vi "InitSubChannel.vi"(9 "GUID":string, 10 "subchannel":i32, 11 "MessengerMCPU in":refnum<class "MessengerMCPU.lvclass">) -> (1 "GUIDsubchannel":i32, 3 "MessengerMCPU out":refnum<class "MessengerMCPU.lvclass">)   [LabVIEW 2019, in "MessengerM.lvlib" / "MessengerMCPU.lvclass"]
uses:
  MessengerMCPU.lvclass
  SubChannelCPU/SubChannelCPU.lvclass
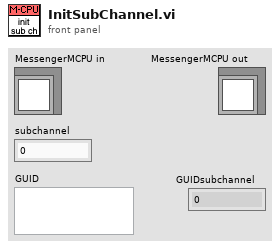
[diagram p1: front panel]
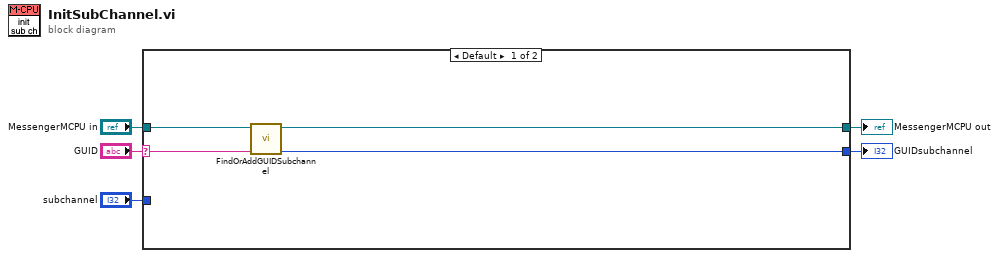
[diagram p0: block diagram]
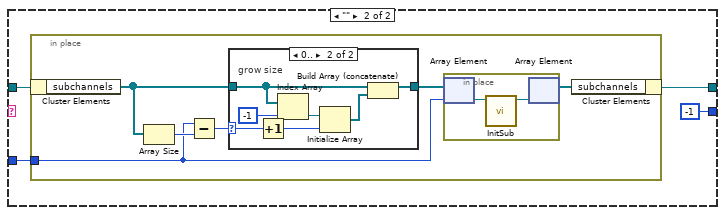
[diagram p2: hidden frame]
diagram:
  n1 = case shown="Default" "GUID" {
    selector: "GUID" -> [w7 _]
    tunnel: "MessengerMCPU in" -> [w9 w13]
    tunnel: [w8 w12] -> w4
    tunnel: "subchannel" -> [_ w11]
    tunnel: [w6 -1 ("GUIDsubchannel")] -> w1
    frame Default {
      n2 = call-dynamic "FindOrAddGUIDSubchannel.vi"("GUID"=w7, "MessengerMCPU in"=w9) -> ("GUIDsubchannel"=w6:i32, "MessengerMCPU out"=w8:refnum<class "MessengerMCPU.lvclass">)  [unwired: 8 in]
    }
    frame "" {
      n3 = in-place {
        in-place-border: w11 -> [w14]
        n4 = in-place-cluster #1(w13) -> ("subchannels"=w17:refnum<class "SubChannelCPU.lvclass">[])
        n5 = Array Size(array=w17) -> (size(s)=w19:i32)
        n6 = Subtract(x=w14, y=w19) -> (x-y=w18:i32)
        n7 = case shown="0.." w18 {
          selector: w18 -> [_ w29]
          tunnel: w17 -> [w22 w26]
          tunnel: [w22 w28] -> w16
          frame Default {
          }
          frame 0.. {
            # "grow size"
            n8 = Increment(x=w29) -> (x+1=w27:i32)
            n9 = Index Array(array=w26, index=-1) -> (element=w24:refnum<class "SubChannelCPU.lvclass">)
            n10 = Initialize Array(w24, w27) -> (w23:refnum<class "SubChannelCPU.lvclass">[])
            n11 = Build Array (concatenate)(w26, w23) -> (w28:refnum<class "SubChannelCPU.lvclass">[])
          }
        }
        n12 = in-place {
          n13 = in-place-array #2(w16, w14) -> (w21:refnum<class "SubChannelCPU.lvclass">)
          n14 = call "InitSub.vi"("SubChannel in"=w21) -> ("SubChannel out"=w20:refnum<class "SubChannelCPU.lvclass">)  [unwired: 10 in]
          n15 = in-place-array #2(w20) -> (w15:refnum<class "SubChannelCPU.lvclass">[])  [unwired: 1 out]
        }
        n16 = in-place-cluster #1("subchannels"=w15) -> (w12:refnum<class "MessengerMCPU.lvclass">)
      }
    }
  }
  "MessengerMCPU out" <- w4
  "GUIDsubchannel" <- w1
